vi "test-Coordinate-axis-Test1.vi"() -> (3 "All tests passed":bool)   [LabVIEW 2019]
uses:
  <vilib>/Rock Robotics/WPI/ThirdParty/JAS_Junk/TrajLib/VI/CoordSystem_New.vi
  <vilib>/Rock Robotics/WPI/ThirdParty/JAS_Junk/TrajLib/Conv_Deg_Radians.vi
  <vilib>/Rock Robotics/WPI/ThirdParty/JAS_Junk/TrajLib/VI/Quaternion_New.vi
  <vilib>/Rock Robotics/WPI/ThirdParty/JAS_Junk/TrajLib/VI/Translation3d_Create.vi
  <vilib>/Rock Robotics/WPI/ThirdParty/JAS_Junk/TrajLib/VI/Pose3d_New_Trans3dRot3d.vi
  <vilib>/Rock Robotics/WPI/ThirdParty/JAS_Junk/TrajLib/VI/Rotation3d_Minus.vi
  <vilib>/Rock Robotics/WPI/ThirdParty/JAS_Junk/TrajLib/VI/Translation3d_Create_Default.vi
  <vilib>/Rock Robotics/WPI/ThirdParty/JAS_Junk/TrajLib/VI/Pose3d_RelativeTo.vi
  <vilib>/Rock Robotics/WPI/ThirdParty/JAS_Junk/TrajLib/VI/Rotation3d_RotateBy.vi
  <vilib>/Rock Robotics/WPI/ThirdParty/JAS_Junk/TrajLib/VI/Translation3d_RotateBy.vi
  <vilib>/Rock Robotics/WPI/ThirdParty/JAS_Junk/TrajLib/VI/Rotation3d_GetQuaterion.vi
  <vilib>/Rock Robotics/WPI/ThirdParty/JAS_Junk/TrajLib/VI/Quaternion_Equals.vi
  <vilib>/Rock Robotics/WPI/ThirdParty/JAS_Junk/TrajLib/VI/CoordAxis_New.vi
  <vilib>/Rock Robotics/WPI/ThirdParty/JAS_Junk/TrajLib/MatBuilder_Create.vi
  <vilib>/Rock Robotics/WPI/ThirdParty/JAS_Junk/TrajLib/Matrix_AssignBlock.vi
  <vilib>/Rock Robotics/WPI/ThirdParty/JAS_Junk/TrajLib/Matrix_Transpose.vi
  <vilib>/Rock Robotics/WPI/ThirdParty/JAS_Junk/TrajLib/Matrix_Ident.vi
  <vilib>/Rock Robotics/WPI/ThirdParty/JAS_Junk/TrajLib/Matrix_IsEqual.vi
  <vilib>/Analysis/baseanly.llb/A x B.vi
  <vilib>/Analysis/baseanly.llb/Real A x B.vi
  <vilib>/Rock Robotics/WPI/ThirdParty/JAS_Junk/TrajLib/VI/Rotation3d_Create_Quaternion.vi
  <vilib>/Rock Robotics/WPI/ThirdParty/JAS_Junk/TrajLib/VI/Rotation3d_UnaryMinus.vi
  <vilib>/Rock Robotics/WPI/ThirdParty/JAS_Junk/TrajLib/VI/Transform3d_Create_Pose3dPose3d.vi
  <vilib>/Rock Robotics/WPI/ThirdParty/JAS_Junk/TrajLib/VI/Transform3d_GetRotation3d.vi
  <vilib>/Rock Robotics/WPI/ThirdParty/JAS_Junk/TrajLib/VI/Transform3d_GetTranslation3d.vi
  <vilib>/Rock Robotics/WPI/ThirdParty/JAS_Junk/TrajLib/VI/Quaternion_Times.vi
  <vilib>/Rock Robotics/WPI/ThirdParty/JAS_Junk/TrajLib/VI/Quaternion_Inverse.vi
  <vilib>/Rock Robotics/WPI/ThirdParty/JAS_Junk/TrajLib/VI/Quaternion_Get_All.vi
  <vilib>/Rock Robotics/WPI/ThirdParty/JAS_Junk/TrajLib/VI/Quaternion_Get_Vect.vi
  <vilib>/Rock Robotics/WPI/ThirdParty/JAS_Junk/TrajLib/VI/Quaternion_Get_W.vi
  <vilib>/Rock Robotics/WPI/ThirdParty/JAS_Junk/TrajLib/MatrixHelper_CoerceSize.vi
  <vilib>/Rock Robotics/WPI/ThirdParty/JAS_Junk/TrajLib/VI/Quaternion_Normalize.vi
  <vilib>/Rock Robotics/WPI/ThirdParty/JAS_Junk/TrajLib/VI/Transform3d_Create_Trans3dRot3d.vi
  <vilib>/Rock Robotics/WPI/ThirdParty/JAS_Junk/TrajLib/VI/Translation3d_Minus.vi
  <vilib>/Rock Robotics/WPI/ThirdParty/JAS_Junk/TrajLib/VI/Quaternion_New_Default.vi
  <vilib>/Analysis/7linalg.llb/Create Special Matrix.vi
  <vilib>/Analysis/7linalg.llb/Create Special Real Matrix.vi
  <vilib>/Analysis/Matrix/Numeric/Conversions/Array To Matrix.vi
  <vilib>/Analysis/Matrix/Numeric/Conversions/Array To Matrix - RA.vi
  <vilib>/Rock Robotics/WPI/ThirdParty/JAS_Junk/TrajLib/Trajectory_Library.lvlib
panel:
  out "Test 4":bool
  out "Test 3":bool
  out "Test 2":bool
  out "Test 1":bool
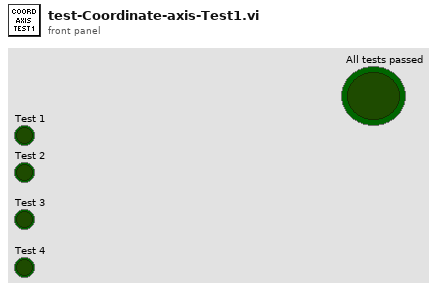
[diagram p1: front panel]
types:
  T1 = typedef "Trajectory_Library.lvlib/ROTATION3D.ctl" = cluster{"Q_quaternion":T2}
  T2 = typedef "Trajectory_Library.lvlib/QUATERNION.ctl" = cluster{"R":dbl, "V":dbl[]}
  T3 = typedef "Trajectory_Library.lvlib/POSE3D.ctl" = cluster{"Translation3d":T4, "Rotation3d":T1}
  T4 = typedef "Trajectory_Library.lvlib/TRANSLATION3D.ctl" = cluster{"X":dbl, "Y":dbl, "Z":dbl}
  T5 = typedef "Trajectory_Library.lvlib/COORDINATE_SYSTEM.ctl" = cluster{"Rotation":T1}
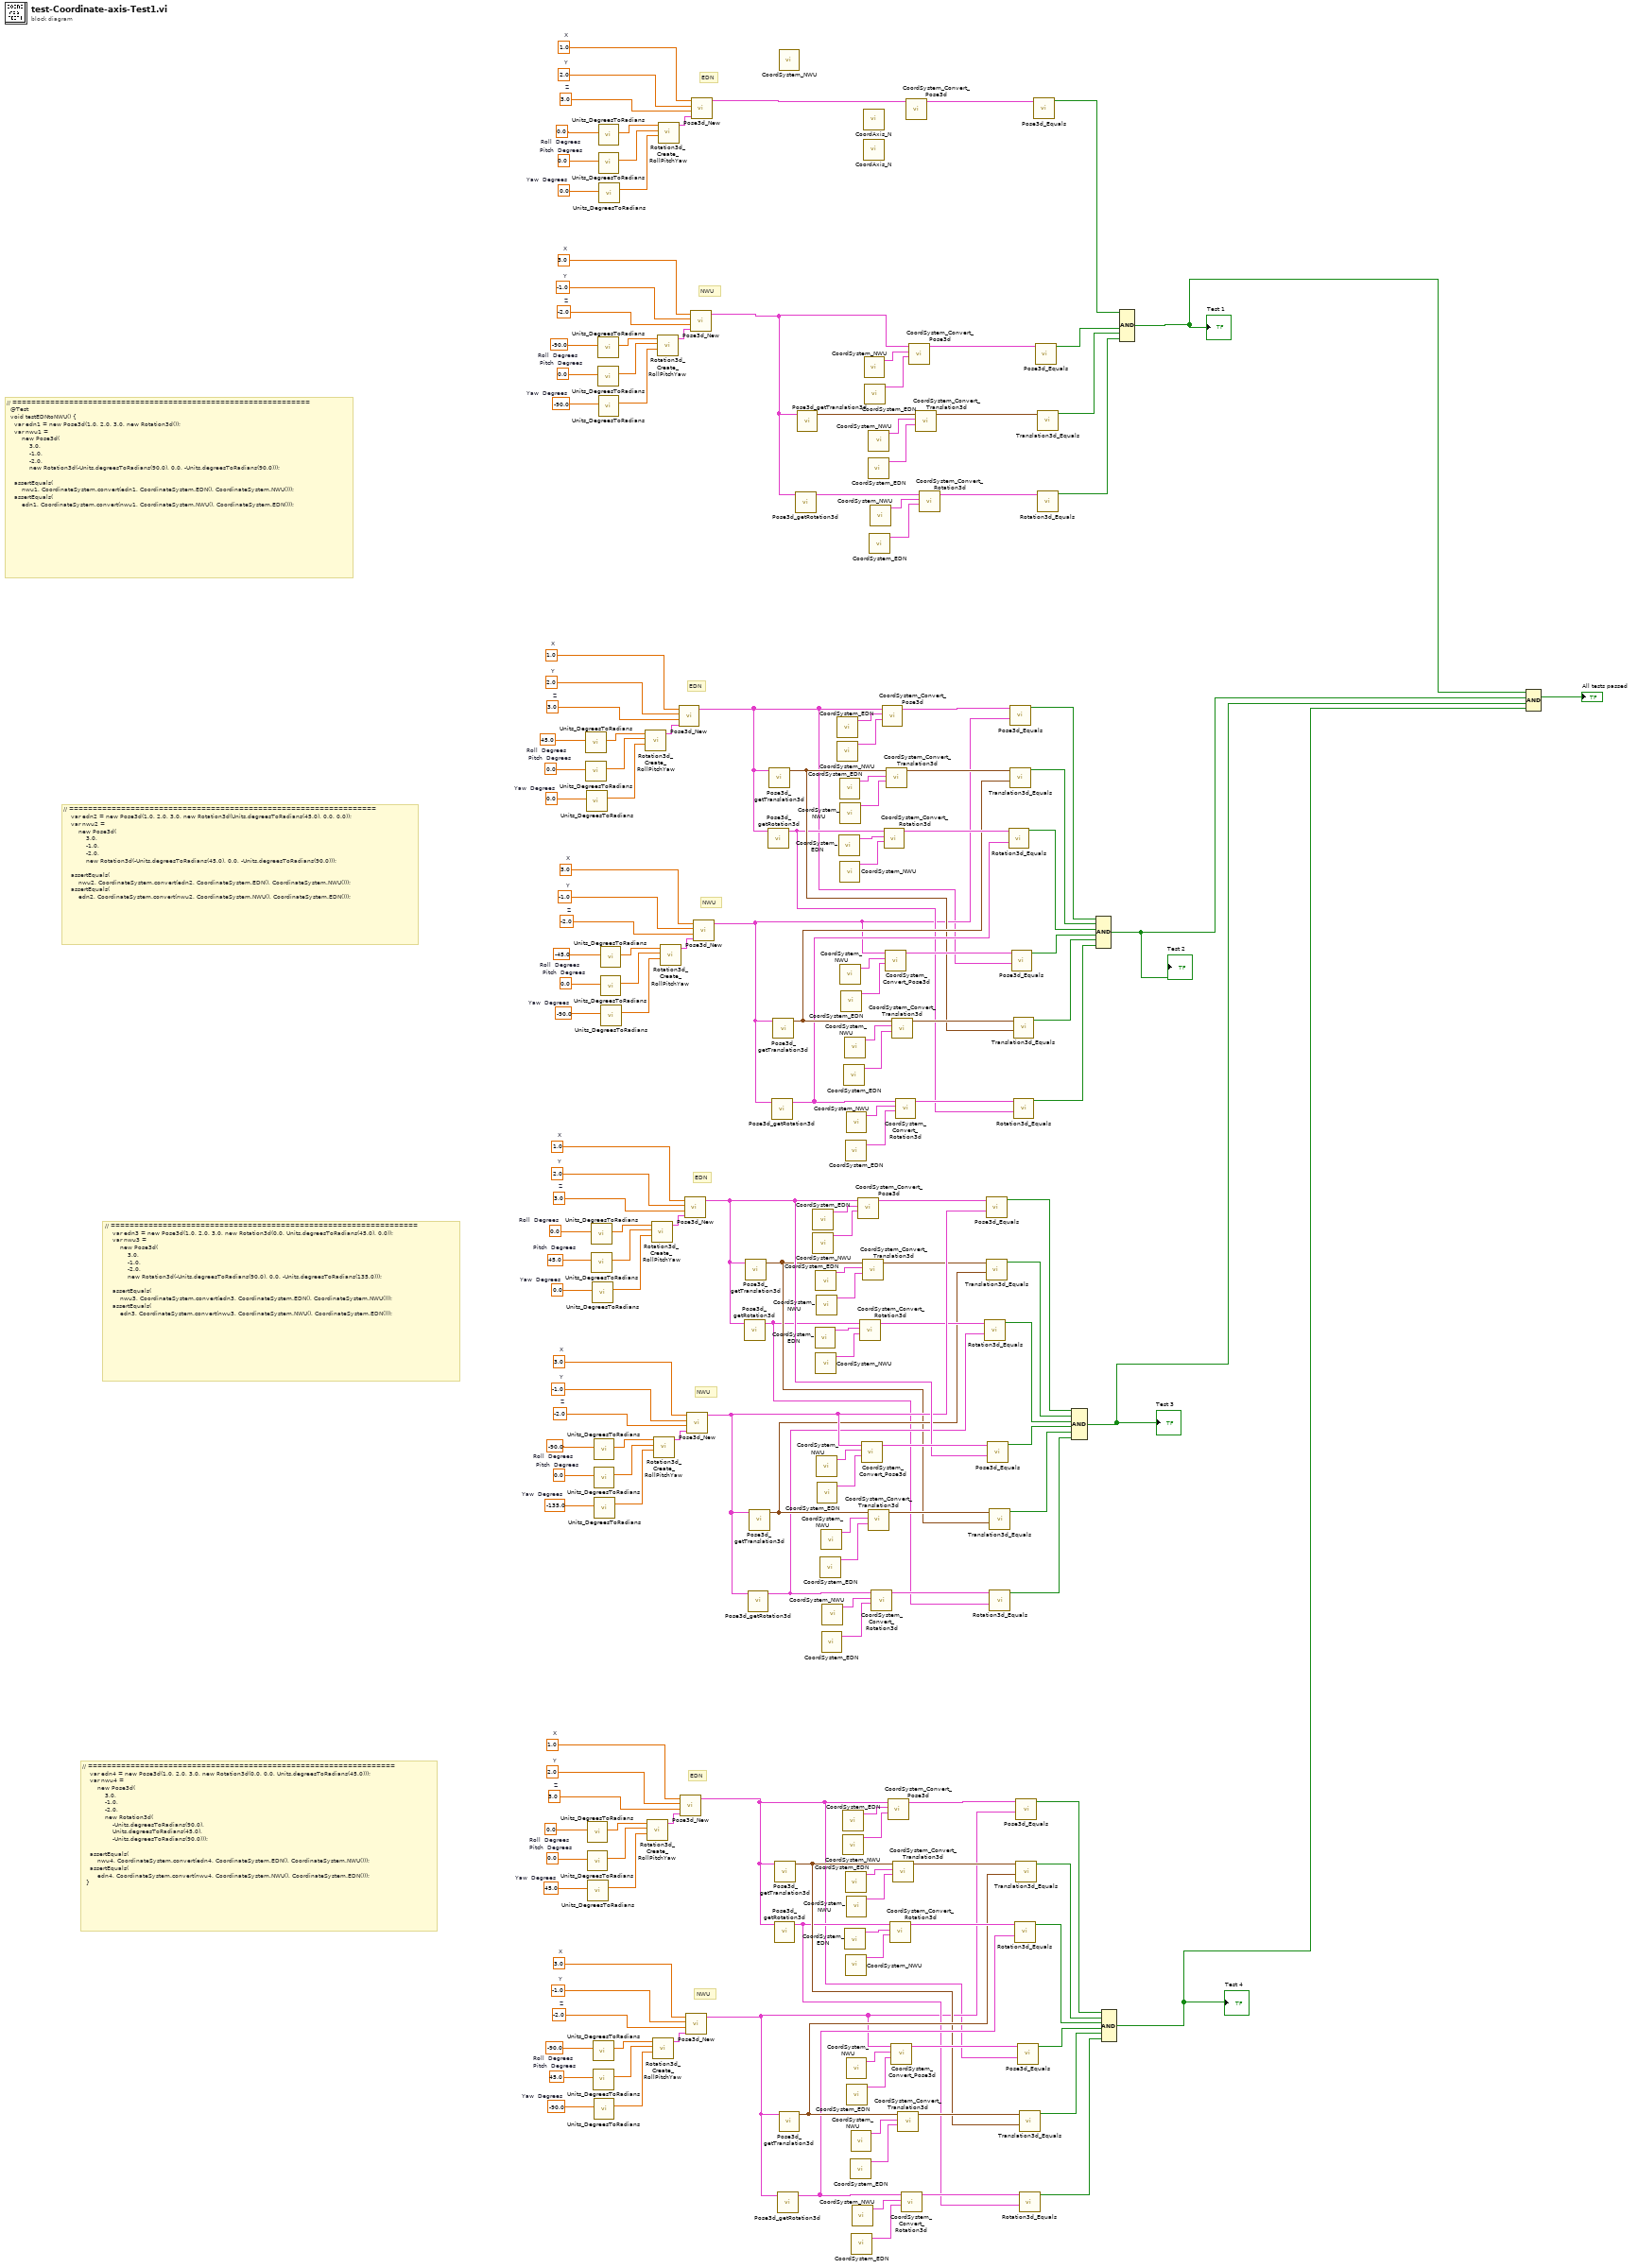
[diagram p0: block diagram]
diagram:
  w114 = 3.0  # X
  w113 = -1.0  # Y
  w112 = -2.0  # Z
  w106 = -90.0  # Roll  Degrees
  w107 = 45.0  # Pitch  Degrees
  w108 = -90.0  # Yaw  Degrees
  w124 = 1.0  # X
  w123 = 2.0  # Y
  w122 = 3.0  # Z
  w116 = 0.0  # Roll  Degrees
  w117 = 0.0  # Pitch  Degrees
  w118 = 45.0  # Yaw  Degrees
  w141 = 3.0  # X
  w140 = -1.0  # Y
  w139 = -2.0  # Z
  w133 = -90.0  # Roll  Degrees
  w134 = 0.0  # Pitch  Degrees
  w135 = -135.0  # Yaw  Degrees
  w151 = 1.0  # X
  w150 = 2.0  # Y
  w149 = 3.0  # Z
  w143 = 0.0  # Roll  Degrees
  w144 = 45.0  # Pitch  Degrees
  w145 = 0.0  # Yaw  Degrees
  w161 = 3.0  # X
  w160 = -1.0  # Y
  w159 = -2.0  # Z
  w153 = -45.0  # Roll  Degrees
  w154 = 0.0  # Pitch  Degrees
  w155 = -90.0  # Yaw  Degrees
  w171 = 1.0  # X
  w170 = 2.0  # Y
  w169 = 3.0  # Z
  w163 = 45.0  # Roll  Degrees
  w164 = 0.0  # Pitch  Degrees
  w165 = 0.0  # Yaw  Degrees
  w182 = 3.0  # X
  w181 = -1.0  # Y
  w180 = -2.0  # Z
  w174 = -90.0  # Roll  Degrees
  w175 = 0.0  # Pitch  Degrees
  w176 = -90.0  # Yaw  Degrees
  w192 = 1.0  # X
  w191 = 2.0  # Y
  w190 = 3.0  # Z
  w184 = 0.0  # Roll  Degrees
  w185 = 0.0  # Pitch  Degrees
  w186 = 0.0  # Yaw  Degrees
  # "// =================================================================\n    var edn2 = new Pose3d(1.0, 2.0, 3.0, new Rotation3d(Units.degreesToRadians(45.0), 0.0, 0.0));\n    var nwu2 =\n        new Pose3d(\n            3.0,\n            -1.0,\n            -2.0,\n            new Rotation3d(-Units.degreesToRadians(45.0), 0.0, -Units.degreesToRadians(90.0)));\n\n    assertEquals(\n        nwu2, CoordinateSystem.convert(edn2, CoordinateSystem.EDN(), CoordinateSystem.NWU()));\n    assertEquals(\n        edn2, CoordinateSystem.convert(nwu2, CoordinateSystem.NWU(), CoordinateSystem.EDN()));"
  # "// =================================================================\n    var edn3 = new Pose3d(1.0, 2.0, 3.0, new Rotation3d(0.0, Units.degreesToRadians(45.0), 0.0));\n    var nwu3 =\n        new Pose3d(\n            3.0,\n            -1.0,\n            -2.0,\n            new Rotation3d(-Units.degreesToRadians(90.0), 0.0, -Units.degreesToRadians(135.0)));\n\n    assertEquals(\n        nwu3, CoordinateSystem.convert(edn3, CoordinateSystem.EDN(), CoordinateSystem.NWU()));\n    assertEquals(\n        edn3, CoordinateSystem.convert(nwu3, CoordinateSystem.NWU(), CoordinateSystem.EDN()));"
  # "// =================================================================\n    var edn4 = new Pose3d(1.0, 2.0, 3.0, new Rotation3d(0.0, 0.0, Units.degreesToRadians(45.0)));\n    var nwu4 =\n        new Pose3d(\n            3.0,\n            -1.0,\n            -2.0,\n            new Rotation3d(\n                -Units.degreesToRadians(90.0),\n                Units.degreesToRadians(45.0),\n                -Units.degreesToRadians(90.0)));\n\n    assertEquals(\n        nwu4, CoordinateSystem.convert(edn4, CoordinateSystem.EDN(), CoordinateSystem.NWU()));\n    assertEquals(\n        edn4, CoordinateSystem.convert(nwu4, CoordinateSystem.NWU(), CoordinateSystem.EDN()));\n  }"
  # "NWU"
  # "EDN"
  # "NWU"
  # "EDN"
  # "NWU"
  # "EDN"
  # "NWU"
  # "EDN"
  # "// ===============================================================\n  @Test\n  void testEDNtoNWU() {\n    var edn1 = new Pose3d(1.0, 2.0, 3.0, new Rotation3d());\n    var nwu1 =\n        new Pose3d(\n            3.0,\n            -1.0,\n            -2.0,\n            new Rotation3d(-Units.degreesToRadians(90.0), 0.0, -Units.degreesToRadians(90.0)));\n\n    assertEquals(\n        nwu1, CoordinateSystem.convert(edn1, CoordinateSystem.EDN(), CoordinateSystem.NWU()));\n    assertEquals(\n        edn1, CoordinateSystem.convert(nwu1, CoordinateSystem.NWU(), CoordinateSystem.EDN()));"
  n1 = call <vilib>:"Units_DegreesToRadians.vi"("Degrees"=w163) -> ("Radians"=w166:dbl)  [unwired: 10 in]
  n2 = call <vilib>:"Units_DegreesToRadians.vi"("Degrees"=w164) -> ("Radians"=w167:dbl)  [unwired: 10 in]
  n3 = call <vilib>:"Units_DegreesToRadians.vi"("Degrees"=w165) -> ("Radians"=w168:dbl)  [unwired: 10 in]
  n4 = call <vilib>:"Units_DegreesToRadians.vi"("Degrees"=w116) -> ("Radians"=w119:dbl)  [unwired: 10 in]
  n5 = call <vilib>:"Units_DegreesToRadians.vi"("Degrees"=w117) -> ("Radians"=w120:dbl)  [unwired: 10 in]
  n6 = call <vilib>:"Units_DegreesToRadians.vi"("Degrees"=w118) -> ("Radians"=w121:dbl)  [unwired: 10 in]
  n7 = call <vilib>:"Units_DegreesToRadians.vi"("Degrees"=w143) -> ("Radians"=w146:dbl)  [unwired: 10 in]
  n8 = call <vilib>:"Units_DegreesToRadians.vi"("Degrees"=w144) -> ("Radians"=w147:dbl)  [unwired: 10 in]
  n9 = call <vilib>:"Units_DegreesToRadians.vi"("Degrees"=w145) -> ("Radians"=w148:dbl)  [unwired: 10 in]
  n10 = call <vilib>:"Units_DegreesToRadians.vi"("Degrees"=w106) -> ("Radians"=w109:dbl)  [unwired: 10 in]
  n11 = call <vilib>:"Units_DegreesToRadians.vi"("Degrees"=w107) -> ("Radians"=w110:dbl)  [unwired: 10 in]
  n12 = call <vilib>:"Units_DegreesToRadians.vi"("Degrees"=w133) -> ("Radians"=w136:dbl)  [unwired: 10 in]
  n13 = call <vilib>:"Units_DegreesToRadians.vi"("Degrees"=w134) -> ("Radians"=w137:dbl)  [unwired: 10 in]
  n14 = call <vilib>:"Units_DegreesToRadians.vi"("Degrees"=w108) -> ("Radians"=w111:dbl)  [unwired: 10 in]
  n15 = call <vilib>:"Units_DegreesToRadians.vi"("Degrees"=w135) -> ("Radians"=w138:dbl)  [unwired: 10 in]
  n16 = call <vilib>:"Units_DegreesToRadians.vi"("Degrees"=w174) -> ("Radians"=w177:dbl)  [unwired: 10 in]
  n17 = call <vilib>:"Units_DegreesToRadians.vi"("Degrees"=w175) -> ("Radians"=w178:dbl)  [unwired: 10 in]
  n18 = call <vilib>:"Units_DegreesToRadians.vi"("Degrees"=w184) -> ("Radians"=w187:dbl)  [unwired: 10 in]
  n19 = call <vilib>:"Units_DegreesToRadians.vi"("Degrees"=w185) -> ("Radians"=w188:dbl)  [unwired: 10 in]
  n20 = call <vilib>:"Units_DegreesToRadians.vi"("Degrees"=w176) -> ("Radians"=w179:dbl)  [unwired: 10 in]
  n21 = call <vilib>:"Units_DegreesToRadians.vi"("Degrees"=w186) -> ("Radians"=w189:dbl)  [unwired: 10 in]
  n22 = call <vilib>:"Units_DegreesToRadians.vi"("Degrees"=w153) -> ("Radians"=w156:dbl)  [unwired: 10 in]
  n23 = call <vilib>:"Units_DegreesToRadians.vi"("Degrees"=w154) -> ("Radians"=w157:dbl)  [unwired: 10 in]
  n24 = call <vilib>:"Units_DegreesToRadians.vi"("Degrees"=w155) -> ("Radians"=w158:dbl)  [unwired: 10 in]
  n25 = call <vilib>:"Rotation3d_Create_RollPitchYaw.vi"("Yaw"=w168, "Pitch"=w167, "Roll"=w166) -> ("Rotation3d"=w172:T1)  [unwired: 8 in]
  n26 = call <vilib>:"Rotation3d_Create_RollPitchYaw.vi"("Yaw"=w121, "Pitch"=w120, "Roll"=w119) -> ("Rotation3d"=w125:T1)  [unwired: 8 in]
  n27 = call <vilib>:"Rotation3d_Create_RollPitchYaw.vi"("Yaw"=w148, "Pitch"=w147, "Roll"=w146) -> ("Rotation3d"=w152:T1)  [unwired: 8 in]
  n28 = call <vilib>:"Rotation3d_Create_RollPitchYaw.vi"("Yaw"=w111, "Pitch"=w110, "Roll"=w109) -> ("Rotation3d"=w115:T1)  [unwired: 8 in]
  n29 = call <vilib>:"Rotation3d_Create_RollPitchYaw.vi"("Yaw"=w138, "Pitch"=w137, "Roll"=w136) -> ("Rotation3d"=w142:T1)  [unwired: 8 in]
  n30 = call <vilib>:"Rotation3d_Create_RollPitchYaw.vi"("Yaw"=w179, "Pitch"=w178, "Roll"=w177) -> ("Rotation3d"=w183:T1)  [unwired: 8 in]
  n31 = call <vilib>:"Rotation3d_Create_RollPitchYaw.vi"("Yaw"=w189, "Pitch"=w188, "Roll"=w187) -> ("Rotation3d"=w193:T1)  [unwired: 8 in]
  n32 = call <vilib>:"Rotation3d_Create_RollPitchYaw.vi"("Yaw"=w158, "Pitch"=w157, "Roll"=w156) -> ("Rotation3d"=w162:T1)  [unwired: 8 in]
  n33 = call <vilib>:"Pose3d_New.vi"("Rotation3d"=w172, "z"=w169, "Y"=w170, "X"=w171) -> ("out Pose3d"=w52:T3)  [unwired: 7 in]
  n34 = call <vilib>:"Pose3d_New.vi"("Rotation3d"=w125, "z"=w122, "Y"=w123, "X"=w124) -> ("out Pose3d"=w2:T3)  [unwired: 7 in]
  n35 = call <vilib>:"Pose3d_New.vi"("Rotation3d"=w152, "z"=w149, "Y"=w150, "X"=w151) -> ("out Pose3d"=w100:T3)  [unwired: 7 in]
  n36 = call <vilib>:"Pose3d_New.vi"("Rotation3d"=w115, "z"=w112, "Y"=w113, "X"=w114) -> ("out Pose3d"=w3:T3)  [unwired: 7 in]
  n37 = call <vilib>:"Pose3d_New.vi"("Rotation3d"=w142, "z"=w139, "Y"=w140, "X"=w141) -> ("out Pose3d"=w99:T3)  [unwired: 7 in]
  n38 = call <vilib>:"Pose3d_New.vi"("Rotation3d"=w183, "z"=w180, "Y"=w181, "X"=w182) -> ("out Pose3d"=w33:T3)  [unwired: 7 in]
  n39 = call <vilib>:"Pose3d_New.vi"("Rotation3d"=w193, "z"=w190, "Y"=w191, "X"=w192) -> ("out Pose3d"=w34:T3)  [unwired: 7 in]
  n40 = call <vilib>:"Pose3d_New.vi"("Rotation3d"=w162, "z"=w159, "Y"=w160, "X"=w161) -> ("out Pose3d"=w53:T3)  [unwired: 7 in]
  n41 = call <vilib>:"Pose3d_getRotation3d.vi"("in Pose3d"=w100) -> ("out Rotation3d"=w87:T1)  [unwired: 10 in]
  n42 = call <vilib>:"Pose3d_getTranslation3d.vi"("in Pose3d"=w100) -> ("out Translation3d"=w88:T4)  [unwired: 10 in]
  n43 = call <vilib>:"Pose3d_getRotation3d.vi"("in Pose3d"=w99) -> ("out Rotation3d"=w89:T1)  [unwired: 10 in]
  n44 = call <vilib>:"Pose3d_getTranslation3d.vi"("in Pose3d"=w99) -> ("out Translation3d"=w90:T4)  [unwired: 10 in]
  n45 = call <vilib>:"Pose3d_getRotation3d.vi"("in Pose3d"=w52) -> ("out Rotation3d"=w59:T1)  [unwired: 10 in]
  n46 = call <vilib>:"Pose3d_getTranslation3d.vi"("in Pose3d"=w52) -> ("out Translation3d"=w60:T4)  [unwired: 10 in]
  n47 = call <vilib>:"Pose3d_getRotation3d.vi"("in Pose3d"=w53) -> ("out Rotation3d"=w61:T1)  [unwired: 10 in]
  n48 = call <vilib>:"Pose3d_getTranslation3d.vi"("in Pose3d"=w53) -> ("out Translation3d"=w62:T4)  [unwired: 10 in]
  n49 = call <vilib>:"Pose3d_getRotation3d.vi"("in Pose3d"=w2) -> ("out Rotation3d"=w9:T1)  [unwired: 10 in]
  n50 = call <vilib>:"Pose3d_getTranslation3d.vi"("in Pose3d"=w2) -> ("out Translation3d"=w10:T4)  [unwired: 10 in]
  n51 = call <vilib>:"Pose3d_getRotation3d.vi"("in Pose3d"=w3) -> ("out Rotation3d"=w11:T1)  [unwired: 10 in]
  n52 = call <vilib>:"CoordSystem_NWU.vi"() -> ()  [unwired: 10 in, 2 out]
  n53 = call <vilib>:"Pose3d_getTranslation3d.vi"("in Pose3d"=w3) -> ("out Translation3d"=w12:T4)  [unwired: 10 in]
  n54 = call <vilib>:"Pose3d_getRotation3d.vi"("in Pose3d"=w33) -> ("out Rotation3d"=w38:T1)  [unwired: 10 in]
  n55 = call <vilib>:"Pose3d_getTranslation3d.vi"("in Pose3d"=w33) -> ("out Translation3d"=w39:T4)  [unwired: 10 in]
  n56 = call <vilib>:"CoordSystem_EDN.vi"() -> ("out Coordinate System"=w132:T5)  [unwired: 10 in, 1 out]
  n57 = call <vilib>:"CoordSystem_NWU.vi"() -> ("out Coordinate System"=w131:T5)  [unwired: 10 in, 1 out]
  n58 = call <vilib>:"CoordSystem_EDN.vi"() -> ("out Coordinate System"=w102:T5)  [unwired: 10 in, 1 out]
  n59 = call <vilib>:"CoordSystem_EDN.vi"() -> ("out Coordinate System"=w104:T5)  [unwired: 10 in, 1 out]
  n60 = call <vilib>:"CoordSystem_NWU.vi"() -> ("out Coordinate System"=w101:T5)  [unwired: 10 in, 1 out]
  n61 = call <vilib>:"CoordSystem_NWU.vi"() -> ("out Coordinate System"=w103:T5)  [unwired: 10 in, 1 out]
  n62 = call <vilib>:"CoordSystem_NWU.vi"() -> ("out Coordinate System"=w130:T5)  [unwired: 10 in, 1 out]
  n63 = call <vilib>:"CoordSystem_EDN.vi"() -> ("out Coordinate System"=w129:T5)  [unwired: 10 in, 1 out]
  n64 = call <vilib>:"CoordSystem_EDN.vi"() -> ("out Coordinate System"=w97:T5)  [unwired: 10 in, 1 out]
  n65 = call <vilib>:"CoordSystem_NWU.vi"() -> ("out Coordinate System"=w98:T5)  [unwired: 10 in, 1 out]
  n66 = call <vilib>:"CoordSystem_EDN.vi"() -> ("out Coordinate System"=w95:T5)  [unwired: 10 in, 1 out]
  n67 = call <vilib>:"CoordSystem_NWU.vi"() -> ("out Coordinate System"=w96:T5)  [unwired: 10 in, 1 out]
  n68 = call <vilib>:"CoordSystem_EDN.vi"() -> ("out Coordinate System"=w81:T5)  [unwired: 10 in, 1 out]
  n69 = call <vilib>:"CoordSystem_NWU.vi"() -> ("out Coordinate System"=w80:T5)  [unwired: 10 in, 1 out]
  n70 = call <vilib>:"CoordSystem_EDN.vi"() -> ("out Coordinate System"=w72:T5)  [unwired: 10 in, 1 out]
  n71 = call <vilib>:"CoordSystem_EDN.vi"() -> ("out Coordinate System"=w74:T5)  [unwired: 10 in, 1 out]
  n72 = call <vilib>:"CoordSystem_NWU.vi"() -> ("out Coordinate System"=w71:T5)  [unwired: 10 in, 1 out]
  n73 = call <vilib>:"CoordSystem_NWU.vi"() -> ("out Coordinate System"=w73:T5)  [unwired: 10 in, 1 out]
  n74 = call <vilib>:"CoordSystem_NWU.vi"() -> ("out Coordinate System"=w79:T5)  [unwired: 10 in, 1 out]
  n75 = call <vilib>:"CoordSystem_EDN.vi"() -> ("out Coordinate System"=w78:T5)  [unwired: 10 in, 1 out]
  n76 = call <vilib>:"CoordSystem_EDN.vi"() -> ("out Coordinate System"=w31:T5)  [unwired: 10 in, 1 out]
  n77 = call <vilib>:"CoordSystem_NWU.vi"() -> ("out Coordinate System"=w30:T5)  [unwired: 10 in, 1 out]
  n78 = call <vilib>:"CoordSystem_EDN.vi"() -> ("out Coordinate System"=w69:T5)  [unwired: 10 in, 1 out]
  n79 = call <vilib>:"CoordSystem_NWU.vi"() -> ("out Coordinate System"=w70:T5)  [unwired: 10 in, 1 out]
  n80 = call <vilib>:"CoordSystem_EDN.vi"() -> ("out Coordinate System"=w22:T5)  [unwired: 10 in, 1 out]
  n81 = call <vilib>:"CoordSystem_EDN.vi"() -> ("out Coordinate System"=w67:T5)  [unwired: 10 in, 1 out]
  n82 = call <vilib>:"CoordSystem_EDN.vi"() -> ("out Coordinate System"=w24:T5)  [unwired: 10 in, 1 out]
  n83 = call <vilib>:"CoordSystem_NWU.vi"() -> ("out Coordinate System"=w21:T5)  [unwired: 10 in, 1 out]
  n84 = call <vilib>:"CoordSystem_NWU.vi"() -> ("out Coordinate System"=w68:T5)  [unwired: 10 in, 1 out]
  n85 = call <vilib>:"CoordSystem_NWU.vi"() -> ("out Coordinate System"=w23:T5)  [unwired: 10 in, 1 out]
  n86 = call <vilib>:"CoordSystem_NWU.vi"() -> ("out Coordinate System"=w29:T5)  [unwired: 10 in, 1 out]
  n87 = call <vilib>:"CoordSystem_EDN.vi"() -> ("out Coordinate System"=w28:T5)  [unwired: 10 in, 1 out]
  n88 = call <vilib>:"CoordSystem_EDN.vi"() -> ("out Coordinate System"=w19:T5)  [unwired: 10 in, 1 out]
  n89 = call <vilib>:"CoordSystem_NWU.vi"() -> ("out Coordinate System"=w20:T5)  [unwired: 10 in, 1 out]
  n90 = call <vilib>:"CoordSystem_EDN.vi"() -> ("out Coordinate System"=w17:T5)  [unwired: 10 in, 1 out]
  n91 = call <vilib>:"CoordSystem_NWU.vi"() -> ("out Coordinate System"=w18:T5)  [unwired: 10 in, 1 out]
  n92 = call <vilib>:"CoordSystem_Convert_Pose3d.vi"("CoordSys To"=w131, "CoordSys From"=w132, "in Pose3d"=w100) -> ("out Converted Pose3d"=w128:T3)  [unwired: 8 in]
  n93 = call <vilib>:"CoordSystem_Convert_Rotation3d.vi"("CoordSys To"=w101, "CoordSys From"=w102, "in Rotation3d"=w87) -> ("out Converted Rotation3d"=w93:T1)  [unwired: 8 in]
  n94 = call <vilib>:"CoordSystem_Convert_Pose3d.vi"("CoordSys To"=w129, "CoordSys From"=w130, "in Pose3d"=w99) -> ("out Converted Pose3d"=w127:T3)  [unwired: 8 in]
  n95 = call <vilib>:"CoordSystem_Convert_Translation3d.vi"("CoordSys To"=w103, "CoordSys From"=w104, "in Translation3d"=w88) -> ("out Converted Translation3d"=w94:T4)  [unwired: 8 in]
  n96 = call <vilib>:"CoordAxis_N.vi"() -> ()  [unwired: 11 in, 1 out]
  n97 = call <vilib>:"CoordAxis_N.vi"() -> ()  [unwired: 11 in, 1 out]
  n98 = call <vilib>:"CoordSystem_NWU.vi"() -> ("out Coordinate System"=w50:T5)  [unwired: 10 in, 1 out]
  n99 = call <vilib>:"CoordSystem_EDN.vi"() -> ("out Coordinate System"=w49:T5)  [unwired: 10 in, 1 out]
  n100 = call <vilib>:"CoordSystem_EDN.vi"() -> ("out Coordinate System"=w44:T5)  [unwired: 10 in, 1 out]
  n101 = call <vilib>:"CoordSystem_Convert_Translation3d.vi"("CoordSys To"=w97, "CoordSys From"=w98, "in Translation3d"=w90) -> ("out Converted Translation3d"=w92:T4)  [unwired: 8 in]
  n102 = call <vilib>:"CoordSystem_NWU.vi"() -> ("out Coordinate System"=w45:T5)  [unwired: 10 in, 1 out]
  n103 = call <vilib>:"CoordSystem_EDN.vi"() -> ("out Coordinate System"=w42:T5)  [unwired: 10 in, 1 out]
  n104 = call <vilib>:"CoordSystem_NWU.vi"() -> ("out Coordinate System"=w43:T5)  [unwired: 10 in, 1 out]
  n105 = call <vilib>:"CoordSystem_Convert_Rotation3d.vi"("CoordSys To"=w95, "CoordSys From"=w96, "in Rotation3d"=w89) -> ("out Converted Rotation3d"=w91:T1)  [unwired: 8 in]
  n106 = call <vilib>:"CoordSystem_Convert_Pose3d.vi"("CoordSys To"=w80, "CoordSys From"=w81, "in Pose3d"=w52) -> ("out Converted Pose3d"=w77:T3)  [unwired: 8 in]
  n107 = call <vilib>:"CoordSystem_Convert_Rotation3d.vi"("CoordSys To"=w71, "CoordSys From"=w72, "in Rotation3d"=w59) -> ("out Converted Rotation3d"=w65:T1)  [unwired: 8 in]
  n108 = call <vilib>:"CoordSystem_Convert_Pose3d.vi"("CoordSys To"=w78, "CoordSys From"=w79, "in Pose3d"=w53) -> ("out Converted Pose3d"=w76:T3)  [unwired: 8 in]
  n109 = call <vilib>:"CoordSystem_Convert_Translation3d.vi"("CoordSys To"=w73, "CoordSys From"=w74, "in Translation3d"=w60) -> ("out Converted Translation3d"=w66:T4)  [unwired: 8 in]
  n110 = call <vilib>:"CoordSystem_Convert_Pose3d.vi"("CoordSys To"=w30, "CoordSys From"=w31, "in Pose3d"=w2) -> ("out Converted Pose3d"=w27:T3)  [unwired: 8 in]
  n111 = call <vilib>:"CoordSystem_Convert_Rotation3d.vi"("CoordSys To"=w21, "CoordSys From"=w22, "in Rotation3d"=w9) -> ("out Converted Rotation3d"=w15:T1)  [unwired: 8 in]
  n112 = call <vilib>:"CoordSystem_Convert_Pose3d.vi"("CoordSys To"=w28, "CoordSys From"=w29, "in Pose3d"=w3) -> ("out Converted Pose3d"=w26:T3)  [unwired: 8 in]
  n113 = call <vilib>:"CoordSystem_Convert_Translation3d.vi"("CoordSys To"=w69, "CoordSys From"=w70, "in Translation3d"=w62) -> ("out Converted Translation3d"=w64:T4)  [unwired: 8 in]
  n114 = call <vilib>:"CoordSystem_Convert_Translation3d.vi"("CoordSys To"=w23, "CoordSys From"=w24, "in Translation3d"=w10) -> ("out Converted Translation3d"=w16:T4)  [unwired: 8 in]
  n115 = call <vilib>:"CoordSystem_Convert_Rotation3d.vi"("CoordSys To"=w67, "CoordSys From"=w68, "in Rotation3d"=w61) -> ("out Converted Rotation3d"=w63:T1)  [unwired: 8 in]
  n116 = call <vilib>:"CoordSystem_Convert_Translation3d.vi"("CoordSys To"=w19, "CoordSys From"=w20, "in Translation3d"=w12) -> ("out Converted Translation3d"=w14:T4)  [unwired: 8 in]
  n117 = call <vilib>:"CoordSystem_Convert_Rotation3d.vi"("CoordSys To"=w17, "CoordSys From"=w18, "in Rotation3d"=w11) -> ("out Converted Rotation3d"=w13:T1)  [unwired: 8 in]
  n118 = call <vilib>:"CoordSystem_Convert_Pose3d.vi"("in Pose3d"=w34) -> ("out Converted Pose3d"=w48:T3)  [unwired: 10 in]
  n119 = call <vilib>:"CoordSystem_Convert_Pose3d.vi"("CoordSys To"=w49, "CoordSys From"=w50, "in Pose3d"=w33) -> ("out Converted Pose3d"=w47:T3)  [unwired: 8 in]
  n120 = call <vilib>:"CoordSystem_Convert_Translation3d.vi"("CoordSys To"=w44, "CoordSys From"=w45, "in Translation3d"=w39) -> ("out Converted Translation3d"=w41:T4)  [unwired: 8 in]
  n121 = call <vilib>:"CoordSystem_Convert_Rotation3d.vi"("CoordSys To"=w42, "CoordSys From"=w43, "in Rotation3d"=w38) -> ("out Converted Rotation3d"=w40:T1)  [unwired: 8 in]
  n122 = call <vilib>:"Rotation3d_Equals.vi"("other Rotation3d"=w89, "in Rotation3d"=w93) -> ("Equals"=w82:bool)  [unwired: 9 in]
  n123 = call <vilib>:"Pose3d_Equals.vi"("other Pose3d"=w99, "in Pose3d"=w128) -> ("Equals"=w84:bool)  [unwired: 9 in]
  n124 = call <vilib>:"Translation3d_Equals.vi"("other Translation3d"=w90, "In Translation3d"=w94) -> ("Equals"=w83:bool)  [unwired: 9 in]
  n125 = call <vilib>:"Pose3d_Equals.vi"("other Pose3d"=w100, "in Pose3d"=w127) -> ("Equals"=w126:bool)  [unwired: 9 in]
  n126 = call <vilib>:"Translation3d_Equals.vi"("other Translation3d"=w88, "In Translation3d"=w92) -> ("Equals"=w86:bool)  [unwired: 9 in]
  n127 = call <vilib>:"Rotation3d_Equals.vi"("other Rotation3d"=w87, "in Rotation3d"=w91) -> ("Equals"=w85:bool)  [unwired: 9 in]
  n128 = call <vilib>:"Rotation3d_Equals.vi"("other Rotation3d"=w61, "in Rotation3d"=w65) -> ("Equals"=w54:bool)  [unwired: 9 in]
  n129 = call <vilib>:"Pose3d_Equals.vi"("other Pose3d"=w53, "in Pose3d"=w77) -> ("Equals"=w56:bool)  [unwired: 9 in]
  n130 = call <vilib>:"Translation3d_Equals.vi"("other Translation3d"=w62, "In Translation3d"=w66) -> ("Equals"=w55:bool)  [unwired: 9 in]
  n131 = call <vilib>:"Pose3d_Equals.vi"("other Pose3d"=w52, "in Pose3d"=w76) -> ("Equals"=w75:bool)  [unwired: 9 in]
  n132 = call <vilib>:"Translation3d_Equals.vi"("other Translation3d"=w60, "In Translation3d"=w64) -> ("Equals"=w58:bool)  [unwired: 9 in]
  n133 = call <vilib>:"Rotation3d_Equals.vi"("other Rotation3d"=w59, "in Rotation3d"=w63) -> ("Equals"=w57:bool)  [unwired: 9 in]
  n134 = call <vilib>:"Rotation3d_Equals.vi"("other Rotation3d"=w11, "in Rotation3d"=w15) -> ("Equals"=w4:bool)  [unwired: 9 in]
  n135 = call <vilib>:"Pose3d_Equals.vi"("other Pose3d"=w3, "in Pose3d"=w27) -> ("Equals"=w6:bool)  [unwired: 9 in]
  n136 = call <vilib>:"Translation3d_Equals.vi"("other Translation3d"=w12, "In Translation3d"=w16) -> ("Equals"=w5:bool)  [unwired: 9 in]
  n137 = call <vilib>:"Pose3d_Equals.vi"("other Pose3d"=w2, "in Pose3d"=w26) -> ("Equals"=w25:bool)  [unwired: 9 in]
  n138 = call <vilib>:"Translation3d_Equals.vi"("other Translation3d"=w10, "In Translation3d"=w14) -> ("Equals"=w8:bool)  [unwired: 9 in]
  n139 = call <vilib>:"Rotation3d_Equals.vi"("other Rotation3d"=w9, "in Rotation3d"=w13) -> ("Equals"=w7:bool)  [unwired: 9 in]
  n140 = call <vilib>:"Pose3d_Equals.vi"("in Pose3d"=w48) -> ("Equals"=w35:bool)  [unwired: 10 in]
  n141 = call <vilib>:"Pose3d_Equals.vi"("in Pose3d"=w47) -> ("Equals"=w46:bool)  [unwired: 10 in]
  n142 = call <vilib>:"Translation3d_Equals.vi"("In Translation3d"=w41) -> ("Equals"=w37:bool)  [unwired: 10 in]
  n143 = call <vilib>:"Rotation3d_Equals.vi"("in Rotation3d"=w40) -> ("Equals"=w36:bool)  [unwired: 10 in]
  n144 = Compound Arithmetic op=AND(w84, w83, w82, w126, w86, w85) -> (w105:bool)
  "Test 3" <- w105
  n145 = Compound Arithmetic op=AND(w56, w55, w54, w75, w58, w57) -> (w51:bool)
  "Test 2" <- w51
  n146 = Compound Arithmetic op=AND(w6, w5, w4, w25, w8, w7) -> (w1:bool)
  "Test 4" <- w1
  n147 = Compound Arithmetic op=AND(w35, w46, w37, w36) -> (w32:bool)  [unwired: 2 in]
  "Test 1" <- w32
  n148 = Compound Arithmetic op=AND(w32, w51, w105, w1) -> (→"All tests passed":bool)
